vi "MGCC_StaEst_testoncomputer.vi"() -> ()   [LabVIEW 2016]
panel:
  out "standard output":string
  in  "Program Path":path=path "%SystemRoot%/System32/calc.exe"
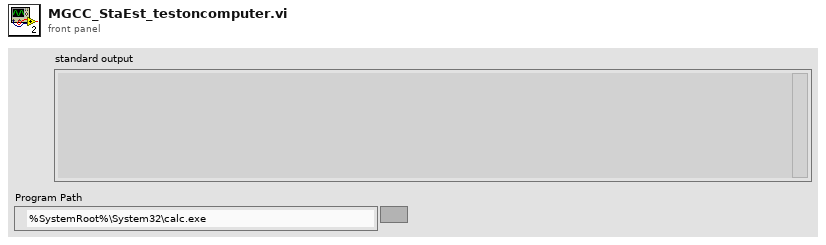
[diagram p1: front panel]
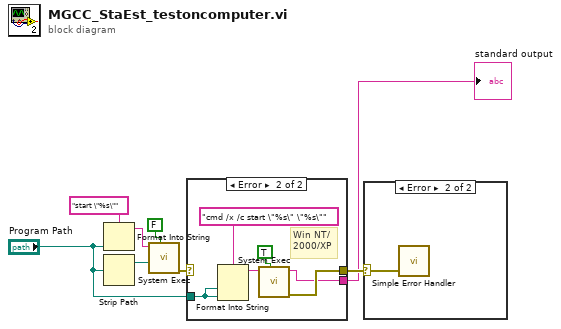
[diagram p0: block diagram]
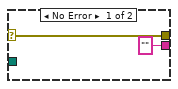
[diagram p3: hidden frame]
diagram:
  n1 = Format Into String(format string="start \"%s\"", "Program Path") -> (resulting string=w4:string)  [unwired: 2 in, 1 out]
  n2 = Strip Path(path="Program Path") -> (stripped path=w5:path)  [unwired: 1 out]
  n3 = call <vilib>:"System Exec.vi"("wait until completion? (T)"=FALSE ("Wait until done"), "working directory"=w5, "command line"=w4) -> ("error out"=w6:errorcluster)  [unwired: 5 in, 3 out]
  n4 = case shown="Error" w6 {
    selector: w6 -> [w10 _]
    tunnel: "Program Path" -> [_ w13]
    tunnel: [w10 w12] -> w8
    tunnel: ["" ("standard output") w11] -> w1
    frame No Error {
    }
    frame Error {
      # "Win NT/\n2000/XP"
      n5 = Format Into String(format string="cmd /x /c start \"%s\" \"%s\"", w13, w13) -> (resulting string=w14:string)  [unwired: 2 in, 1 out]
      n6 = call <vilib>:"System Exec.vi"("wait until completion? (T)"=TRUE ("Wait until done"), "command line"=w14) -> ("error out"=w12:errorcluster, "standard output"=w11:string)  [unwired: 6 in, 2 out]
    }
  }
  "standard output" <- w1
  n7 = case shown="Error" w8 {
    selector: w8 -> [_ w17]
    frame No Error {
    }
    frame Error {
      n8 = call <vilib>:"Simple Error Handler.vi"("error in (no error)"=w17) -> ()  [unwired: 4 in, 5 out]
    }
  }
